vi "User Console - Fire Transactions.vi"(8 "error in (no error)":errorcluster, 10 "Transaction Enum":T2, 11 "UE Data Container":T1) -> (0 "error out":errorcluster, 3 "UE Data Container":T1)   [LabVIEW 2017]
doc: "Generates User Event when any transaction is pressed."
uses:
  Controls/User Console - Transaction Enum.ctl
  Shared Data/User Events/UE Data Container.ctl
  Error Handler/Controls/Error Data.ctl
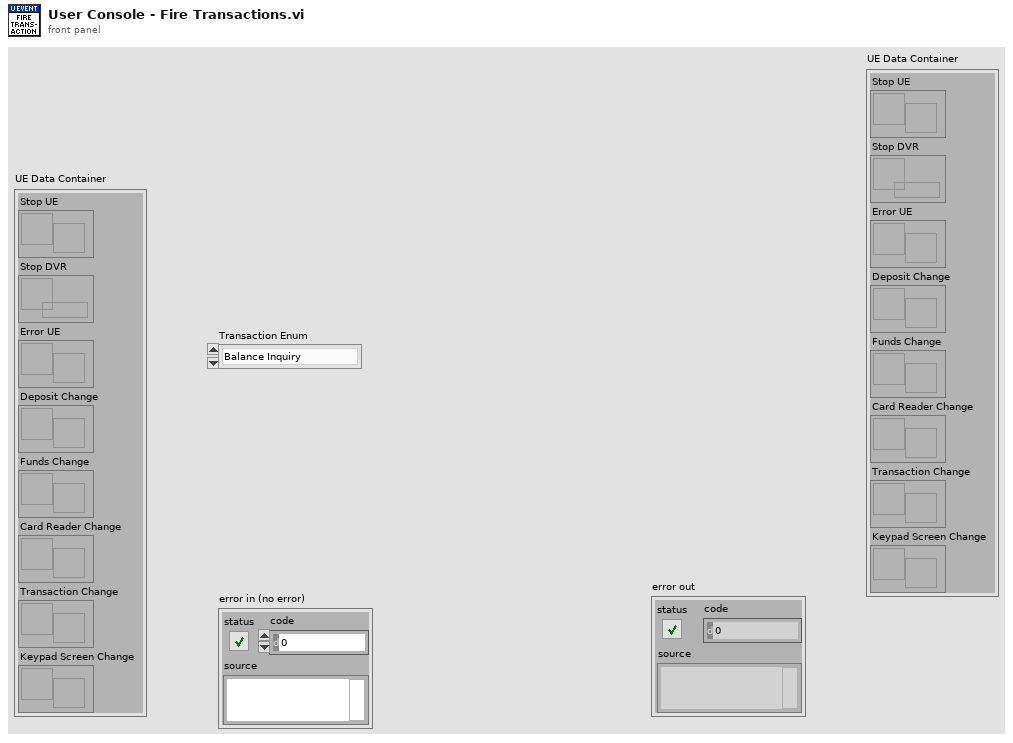
[diagram p1: front panel]
types:
  T1 = typedef "UE Data Container.ctl" = cluster{"Stop UE":refnum<user-event>, "Stop DVR":refnum<data-value>, "Error UE":refnum<user-event>, "Deposit Change":refnum<user-event>, "Funds Change":refnum<user-event>, "Card Reader Change":refnum<user-event>, "Transaction Change":refnum<user-event>, "Keypad Screen Change":refnum<user-event>}
  T2 = typedef "User Console - Transaction Enum.ctl" = enum16{"Balance Inquiry", "Deposit", "Withdrawal", "Fat Cash", "New Transaction", "Terminate Session"}
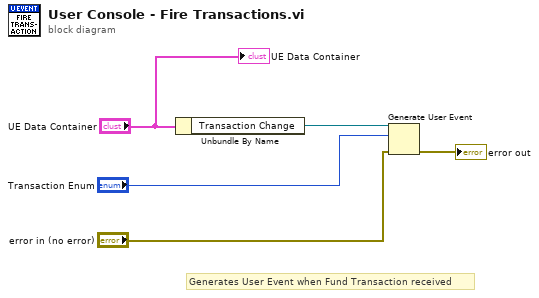
[diagram p0: block diagram]
diagram:
  # "Generates User Event when Fund Transaction received"
  n1 = Unbundle By Name("UE Data Container") -> ("Transaction Change"=w5:refnum<user-event>)
  n2 = Generate User Event(user event=w5, event data cluster="Transaction Enum", error in="error in (no error)") -> (error out=→"error out":errorcluster)  [unwired: 1 in, 1 out]
  "UE Data Container" <- "UE Data Container"
